vi "Read Ref No_.vi"(8 "error in (no error)":errorcluster, 11 "AlessiRel6100 in":refnum<class "AlessiRel6100.lvclass">) -> (0 "error out":errorcluster, 2 "Ref No.":u32, 3 "AlessiRel6100 out":refnum<class "AlessiRel6100.lvclass">)   [LabVIEW 2019, in "AlessiRel6100.lvclass"]
uses:
  AlessiRel6100.lvclass
  AlessiRel6100.lvclass/AlessiRel6100.ctl
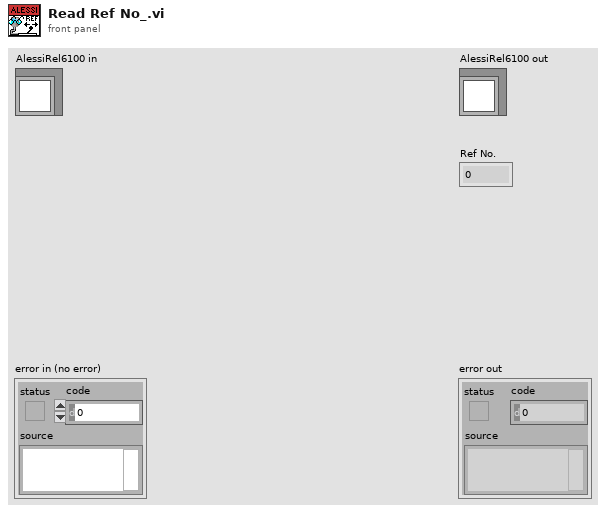
[diagram p1: front panel]
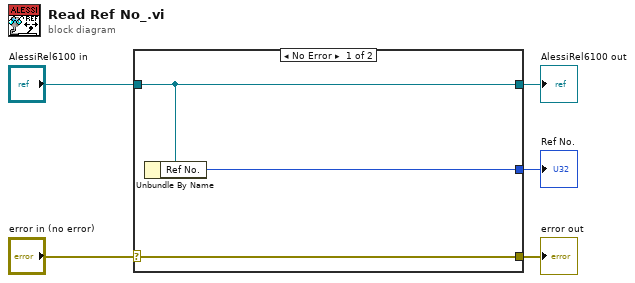
[diagram p0: block diagram]
diagram:
  n1 = case shown="No Error" "error in (no error)" {
    selector: "error in (no error)" -> [w8 w9]
    tunnel: [w8 w9] -> w4
    tunnel: [w7 w10] -> w2
    tunnel: "AlessiRel6100 in" -> [w7 w10]
    tunnel: [w6 _] -> w1
    frame No Error {
      n2 = Unbundle By Name(w7) -> ("Ref No."=w6:u32)
    }
    frame Error {
    }
  }
  "error out" <- w4
  "AlessiRel6100 out" <- w2
  "Ref No." <- w1
